vi "Test2.vi"() -> ()   [LabVIEW 2017]
panel:
  in  "String":string
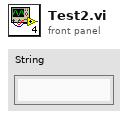
[diagram p1: front panel]
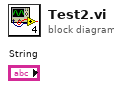
[diagram p0: block diagram]
diagram:
